vi "CheckMouseClicks.vi"(0 "Mouse":T1, 1 "Boundaries":cluster{"low":i32, "high":i32}[](array[cluster])=[{"low"=10, "high"=22}, {"low"=30, "high"=42}, {"low"=50, "high"=62}]) -> (2 "Change?":bool, 3 "Shift?":bool, 4 "selection":i32)   [LabVIEW 2015]
uses:
  vi.lib/Utility/miscctls.llb/LVMouseTypeDef.ctl
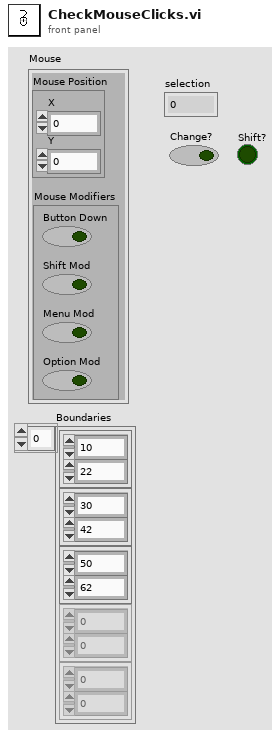
[diagram p1: front panel]
types:
  T1 = typedef "LVMouseTypeDef.ctl" = cluster{"Mouse Position":cluster{"X":i32, "Y":i32}, "Mouse Modifiers":cluster{"Button Down":bool, "Shift Mod":bool, "Menu Mod":bool, "Option Mod":bool}}
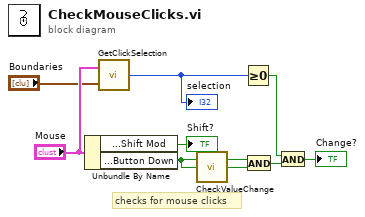
[diagram p0: block diagram]
diagram:
  # "checks for mouse clicks"
  n1 = Unbundle By Name("Mouse") -> ("Mouse Modifiers.Shift Mod"=→"Shift?":bool, "Mouse Modifiers.Button Down"=w8:bool)
  n2 = call "GetClickSelection.vi"("Boundaries"="Boundaries", "Mouse"="Mouse") -> ("selection"=w3:i32)
  "selection" <- w3
  n3 = call "CheckValueChange.vi"("Button Down"=w8) -> ("Boolean"=w7:bool)
  n4 = Greater Or Equal To 0?(x=w3) -> (x >= 0?=w6:bool)
  n5 = And(x=w8, y=w7) -> (x .and. y?=w5:bool)
  n6 = And(x=w6, y=w5) -> (x .and. y?=→"Change?":bool)
